vi "Create Zero Plane.vi"(7 "3D Mesh Property":T4={"General Property"={"Plot Name"="", "Coordinate System"=enum."Cartesian", "Opacity"=0.0}, "Projection Property"={"Draw XY"=FALSE, "Draw YZ"=FALSE, "Draw XZ"=FALSE}, "Plot Property"={"Surface Color"=0, "Line Style"=enum."None", "Line Width"=0.0, "Color Ramp Cluster"={"Color Ramp Style"=enum."None", "Color Ramp Array"=[16711934, 393471, 57855, 4390754, 16449346, 16744722, 16711680], "Color Ramp Index"=[45, 91, 133, 175, 219, 255], "Interpolate?"=FALSE, "Logarithm?"=FALSE}, "Antialiasing"=FALSE}, "Mesh Property"={"Mesh Mode"=enum."Lines"}}, 8 "error in (no error)":errorcluster, 9 "Actual Transform In":T7, 10 "Plot Representation In":T1, 11 "Plot Object In":refnum<vi>) -> (0 "error out":errorcluster, 1 "Actual Transform Out":T7, 2 "Plot Representation Out":T1, 3 "Plot Object Out":refnum<vi>, 4 "Zero Plane Object Out":refnum<vi>)   [LabVIEW 2017, in "3D Mesh.lvclass"]
uses:
  <vilib>/Math Plots/3D Math Plots/3D Mesh/3D Mesh/3D Mesh.lvclass
  <vilib>/Math Plots/3D Math Plots/3D Plot/3D Plot/Typedef/Actual Transform.ctl
  <vilib>/Math Plots/3D Math Plots/3D Plot/3D Plot/Typedef/Range Clusters.ctl
  <vilib>/Math Plots/3D Math Plots/3D Plot/3D Plot/Typedef/Plot Representation.ctl
  <vilib>/Math Plots/3D Math Plots/3D Plot/3D Plot/Typedef/Mesh Data.ctl
  <vilib>/Math Plots/3D Math Plots/3D Mesh/3D Mesh/Typedef/3D Mesh Property.ctl
  <vilib>/Math Plots/3D Math Plots/3D Plot/3D Plot/Typedef/Line Type.ctl
  <vilib>/Math Plots/3D Math Plots/3D Plot/3D Plot/Typedef/Color Ramp Cluster.ctl
  <vilib>/picture/3D Picture Control/Object/Create Object (name).vi
  <vilib>/picture/3D Picture Control/NI_3D Picture Control.lvlib
  <vilib>/Math Plots/3D Math Plots/3D Plot/3D Plot/3D Plot.lvclass
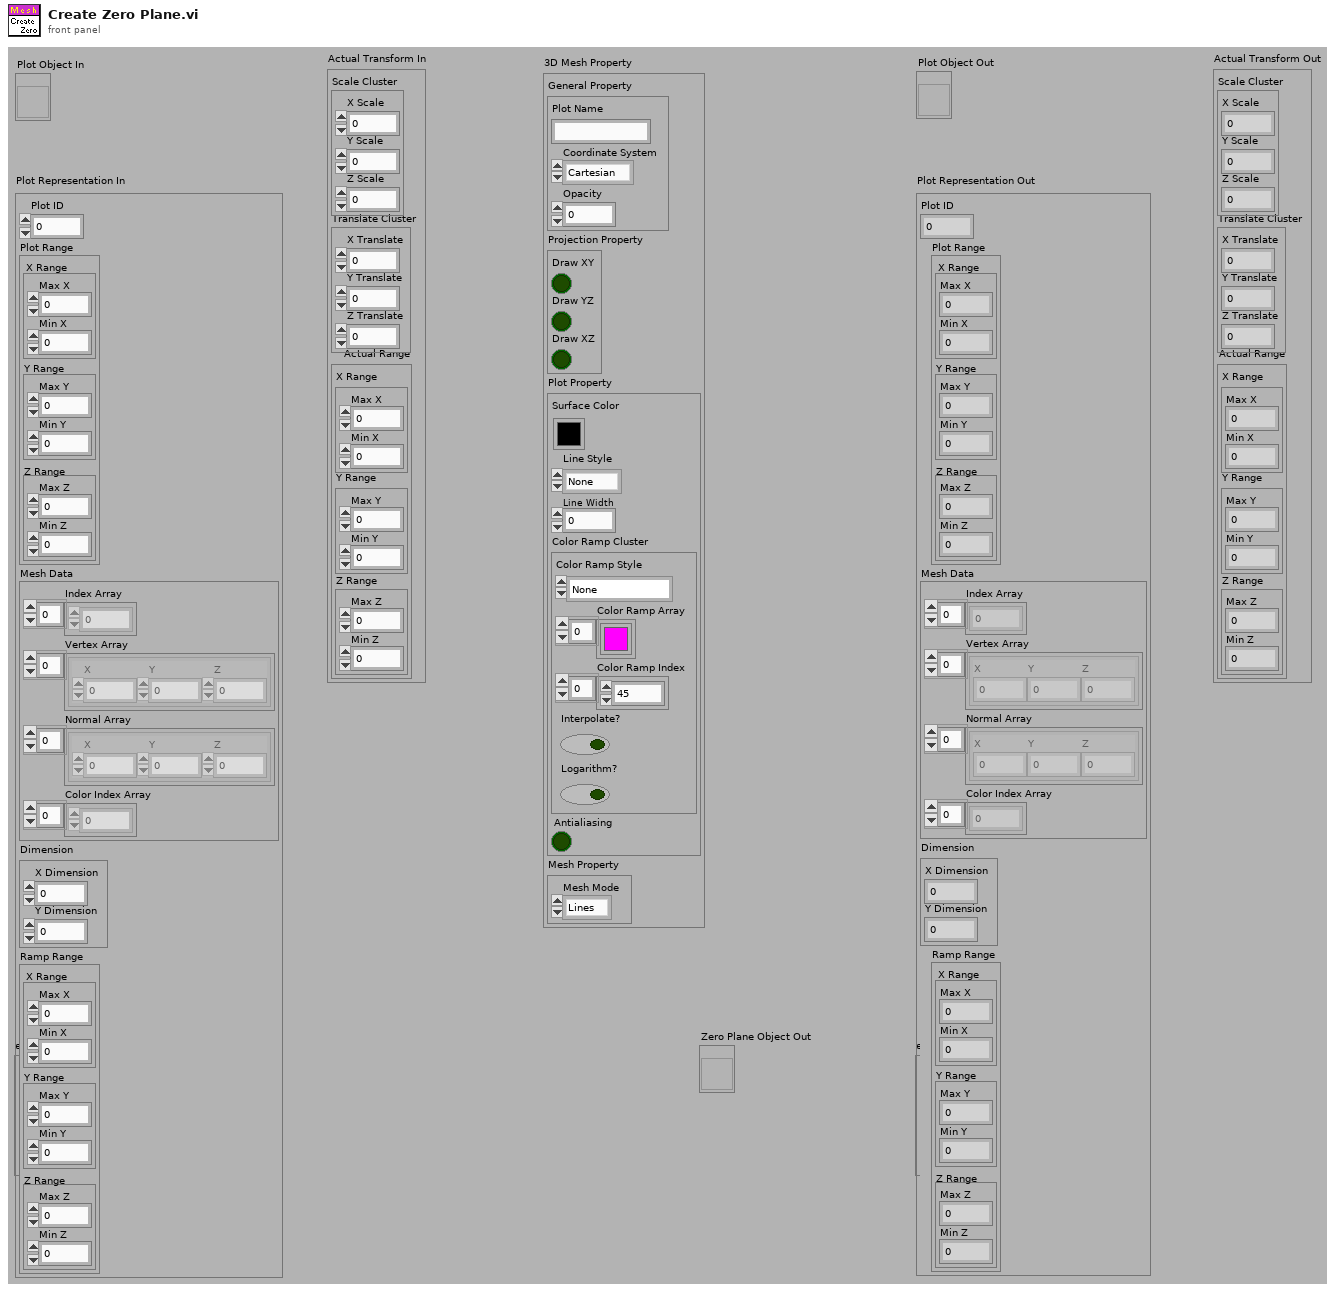
[diagram p1: front panel]
types:
  T1 = typedef "3D Plot.lvclass/Plot Representation.ctl" = cluster{"Plot ID":i32, "Plot Range":T2, "Mesh Data":T3, "Dimension":cluster{"X Dimension":i32, "Y Dimension":i32}, "Ramp Range":T2}
  T2 = typedef "3D Plot.lvclass/Range Clusters.ctl" = cluster{"X Range":cluster{"Max X":sgl, "Min X":sgl}, "Y Range":cluster{"Max Y":sgl, "Min Y":sgl}, "Z Range":cluster{"Max Z":sgl, "Min Z":sgl}}
  T3 = typedef "3D Plot.lvclass/Mesh Data.ctl" = cluster{"Index Array":u32[], "Vertex Array":cluster{"X":sgl, "Y":sgl, "Z":sgl}[], "Normal Array":cluster{"X":sgl, "Y":sgl, "Z":sgl}[], "Color Index Array":i32[]}
  T4 = typedef "3D Mesh.lvclass/3D Mesh Property.ctl" = cluster{"General Property":cluster{"Plot Name":string, "Coordinate System":enum16{"Cartesian", "Cylindrical", "Spherical"}, "Opacity":sgl}, "Projection Property":cluster{"Draw XY":bool, "Draw YZ":bool, "Draw XZ":bool}, "Plot Property":cluster{"Surface Color":u32, "Line Style":T5, "Line Width":sgl, "Color Ramp Cluster":T6, "Antialiasing":bool}, "Mesh Property":cluster{"Mesh Mode":enum16{"Lines", "Hidden Lines", "With Zero Plane"}}}
  T5 = typedef "3D Plot.lvclass/Line Type.ctl" = enum16{"None", "Solid", "Dash", "Dot", "Dash Dot"}
  T6 = typedef "3D Plot.lvclass/Color Ramp Cluster.ctl" = cluster{"Color Ramp Style":enum16{"None", "Shaded", "Color spectrum", "Grey scale", "Custom"}, "Color Ramp Array":u32[], "Color Ramp Index":i32[], "Interpolate?":bool, "Logarithm?":bool}
  T7 = typedef "3D Plot.lvclass/Actual Transform.ctl" = cluster{"Scale Cluster":cluster{"X Scale":sgl, "Y Scale":sgl, "Z Scale":sgl}, "Translate Cluster":cluster{"X Translate":sgl, "Y Translate":sgl, "Z Translate":sgl}, "Actual Range":T2}
  T8 = enum16{"Overall", "Per Primitive", "Per Vertex", "Binding Off"}
  T9 = enum16{"Points", "Lines", "Line Strip", "Line Loop", "Triangles", "Triangle Strip", "Triangle Fan", "Quads", "Quad Strip", "Polygon"}
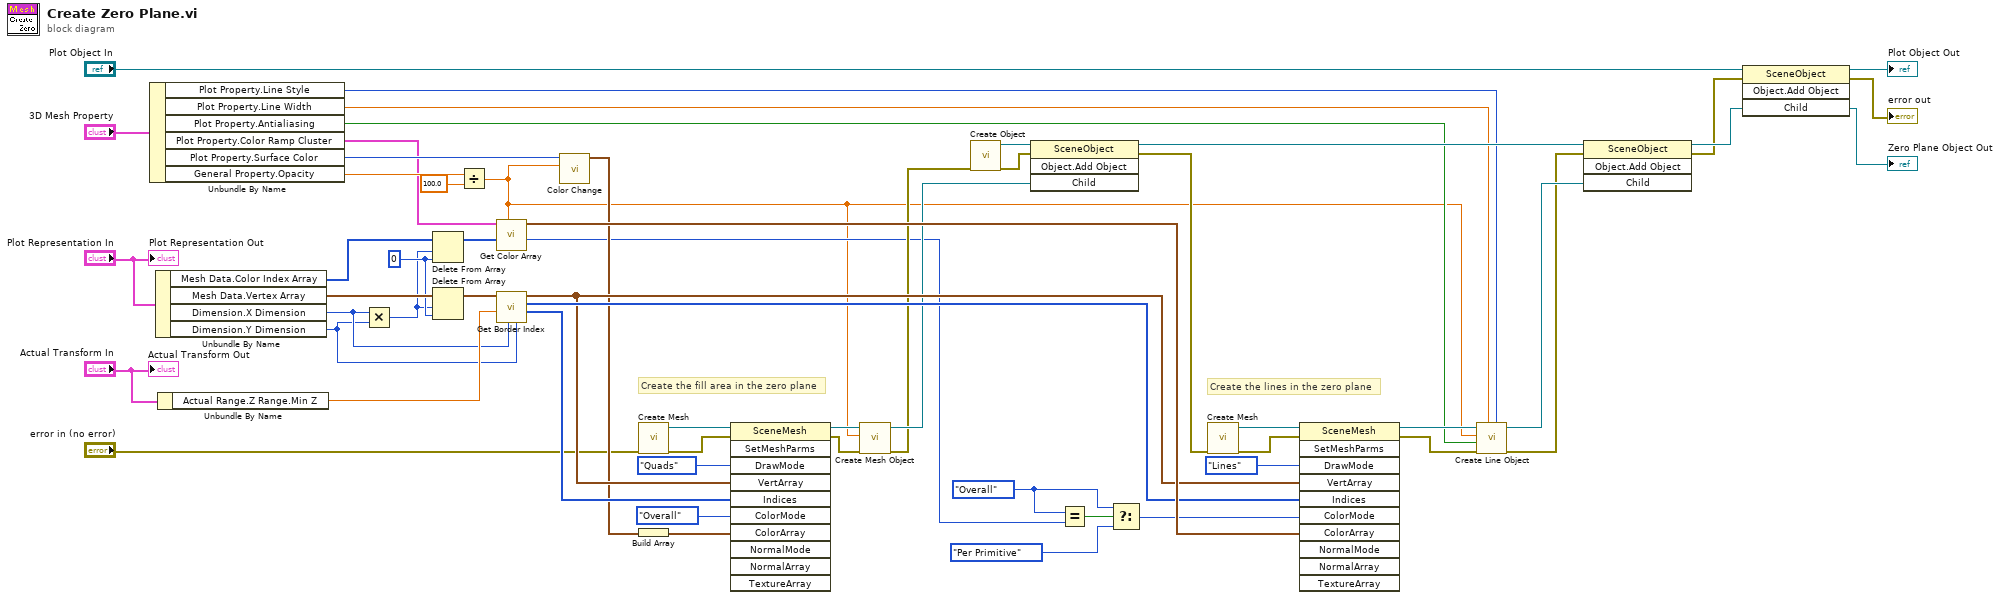
[diagram p0: block diagram]
diagram:
  w2 = 0 ("index")
  w13 = T8."Overall" ("y")
  # "Create the lines in the zero plane"
  # "Create the fill area in the zero plane"
  n1 = Unbundle By Name("3D Mesh Property") -> ("Plot Property.Line Style"=w11:T5, "Plot Property.Line Width"=w12:sgl, "Plot Property.Antialiasing"=w10:bool, "Plot Property.Color Ramp Cluster"=w7:T6, "Plot Property.Surface Color"=w31:u32, "General Property.Opacity"=w8:sgl)
  n2 = Unbundle By Name("Plot Representation In") -> ("Mesh Data.Color Index Array"=w6:i32[], "Mesh Data.Vertex Array"=w4:cluster{"X":sgl, "Y":sgl, "Z":sgl}[], "Dimension.X Dimension"=w43:i32, "Dimension.Y Dimension"=w42:i32)
  n3 = Unbundle By Name("Actual Transform In") -> ("Actual Range.Z Range.Min Z"=w48:sgl)
  n4 = Multiply(x=w43, y=w42) -> (x*y=w1:i32)
  n5 = Delete From Array(array=w6, length=w1, index=w2) -> (array with subset deleted=w5:i32[])  [unwired: 1 out]
  n6 = Delete From Array(array=w4, length=w1, index=w2) -> (array with subset deleted=w3:cluster{"X":sgl, "Y":sgl, "Z":sgl}[])  [unwired: 1 out]
  n7 = Divide(x=w8, y=sgl 100.0) -> (x/y=w9:sgl)
  n8 = call <vilib>:"Get Color Array.vi"("Alpha"=w9, "Color Index Array"=w5, "Color Ramp Cluster"=w7) -> ("Color Binding Mode"=w17:T8, "Color Array"=w51:cluster{"R":sgl, "G":sgl, "B":sgl, "A":sgl}[])  [unwired: 4 in, 3 out]
  n9 = call <vilib>:"Get Border Index.vi"("Y Dimension"=w42, "X Dimension"=w43, "Min Z"=w48, "Border Vertex Array In"=w3) -> ("Polygens Index Array"=w34:u32[], "Wireframe Index Array"=w49:u32[], "Border Vertex Array Out"=w35:cluster{"X":sgl, "Y":sgl, "Z":sgl}[])  [unwired: 5 out]
  n10 = call <vilib>:"Color Change.vi"("Alpha"=w9, "Color"=w31) -> ("RGBA"=w33:cluster{"R":sgl, "G":sgl, "B":sgl, "A":sgl})  [unwired: 9 out]
  n11 = call <vilib>:"Create Mesh.vi"("error in (no error)"="error in (no error)") -> ("error out"=w39:errorcluster, "New Mesh Refnum"=w38:refnum<vi>)  [unwired: 9 out]
  n12 = Build Array(w33) -> (w32:cluster{"R":sgl, "G":sgl, "B":sgl, "A":sgl}[])
  n13 = invoke class="SceneMesh" method="SetMeshParms"(reference=w38, error in=w39, "DrawMode"=T9."Quads" ("Draw Mode"), "VertArray"=w35, "Indices"=w34, "ColorMode"=T8."Overall" ("Color Binding Mode"), "ColorArray"=w32) -> (reference out=w37:refnum<vi>, error out=w36:errorcluster)  [unwired: 4 in, 9 out]
  n14 = call <vilib>:"Create Mesh Object.vi"("error in (no error)"=w36, "Alpha"=w9, "Mesh Object In"=w37) -> ("error out"=w21:errorcluster, "Object Ref Out"=w29:refnum<vi>)  [unwired: 1 in, 6 out]
  n15 = call-poly <vilib>:"Create Object.vi"("error in (no error)"=w21) -> ("error out"=w20:errorcluster, "Scene:New Object"=w26:refnum<vi>)  [unwired: 9 in]
  n16 = invoke class="SceneObject" method="Object.Add Object"(reference=w26, error in=w20, "Child"=w29) -> (reference out=w30:refnum<vi>, error out=w27:errorcluster)  [unwired: 1 in, 2 out]
  n17 = Equal?(x=w13, y=w17) -> (x = y?=w16:bool)
  n18 = Select(t=w13, s=w16, f=T8."Per Primitive" ("Color Binding Mode")) -> (s? t:f=w14:T8)
  n19 = call <vilib>:"Create Mesh.vi"("error in (no error)"=w27) -> ("error out"=w53:errorcluster, "New Mesh Refnum"=w54:refnum<vi>)  [unwired: 9 out]
  n20 = invoke class="SceneMesh" method="SetMeshParms"(reference=w54, error in=w53, "DrawMode"=T9."Lines" ("Draw Mode"), "VertArray"=w35, "Indices"=w49, "ColorMode"=w14, "ColorArray"=w51) -> (reference out=w47:refnum<vi>, error out=w46:errorcluster)  [unwired: 4 in, 9 out]
  n21 = call <vilib>:"Create Line Object.vi"("Line Style"=w11, "Line Width"=w12, "error in (no error)"=w46, "Antialiasing"=w10, "Alpha"=w9, "Mesh Ref In"=w47) -> ("error out"=w44:errorcluster, "Object Ref Out"=w45:refnum<vi>)  [unwired: 4 out]
  n22 = invoke class="SceneObject" method="Object.Add Object"(reference=w30, error in=w44, "Child"=w45) -> (reference out=w25:refnum<vi>, error out=w19:errorcluster)  [unwired: 1 in, 2 out]
  n23 = invoke class="SceneObject" method="Object.Add Object"(reference="Plot Object In", error in=w19, "Child"=w25) -> (reference out=→"Plot Object Out":refnum<vi>, error out=→"error out":errorcluster, "Child"=→"Zero Plane Object Out":refnum<vi>)  [unwired: 1 in, 1 out]
  "Actual Transform Out" <- "Actual Transform In"
  "Plot Representation Out" <- "Plot Representation In"
